vi "getMethods.vi"(0 "reference in":refnum<class "DQMHModuleNode.lvclass">, 5 "error in (no error)":errorcluster) -> (14 "reference out":refnum<class "DQMHModuleNode.lvclass">, 15 "methods":refnum<class "MultiLineString.lvclass">, 19 "error out":errorcluster)   [LabVIEW 2014, in "DQMHModuleNode.lvclass"]
doc: "public MultiLineString getMethods()"
uses:
  <resource>/Framework/Providers/Open_GDS/UML/DQMHModuleNode_class/DQMHModuleNode.lvclass
  <resource>/Framework/Providers/Open_GDS/UML/MultiLineString_class/MultiLineString.lvclass
panel:
  # "Always set\nVI Server class\nto current VI. Do not\nconnect this control\nto the connector pane.\n(Tip!: Just drag\nand drop the icon\ninto the refnum)"
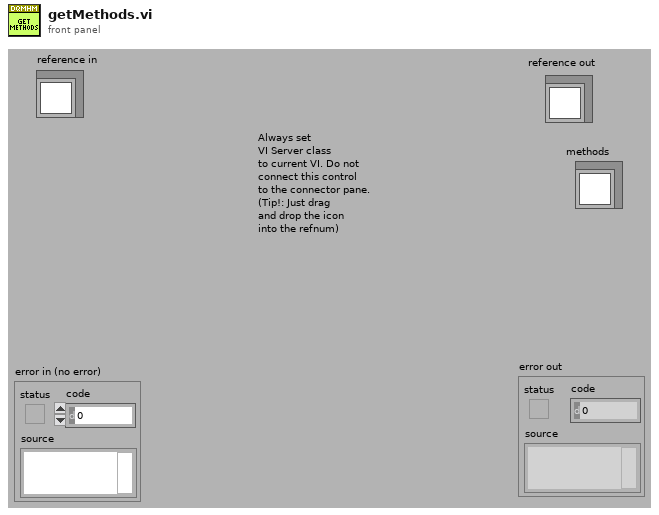
[diagram p1: front panel]
types:
  T1 = typedef "DQMHModuleNode.lvclass/ObjectAttributes.ctl" = cluster{"midHeight":dbl, "botHeight":dbl, "Name":refnum<class "MultiLineString.lvclass">, "Description":refnum<class "MultiLineString.lvclass">, "InternalData":refnum<class "MultiLineString.lvclass">, "Events":refnum<class "MultiLineString.lvclass">, "DEFAULT_COMPARTMENT_HEIGHT":i32, "DEFAULT_WIDTH":i32, "DEFAULT_HEIGHT":i32, "showEvents":bool, "showInternalData":bool, "ClassPath":path, "Template":string, "Icon":u8[][]}
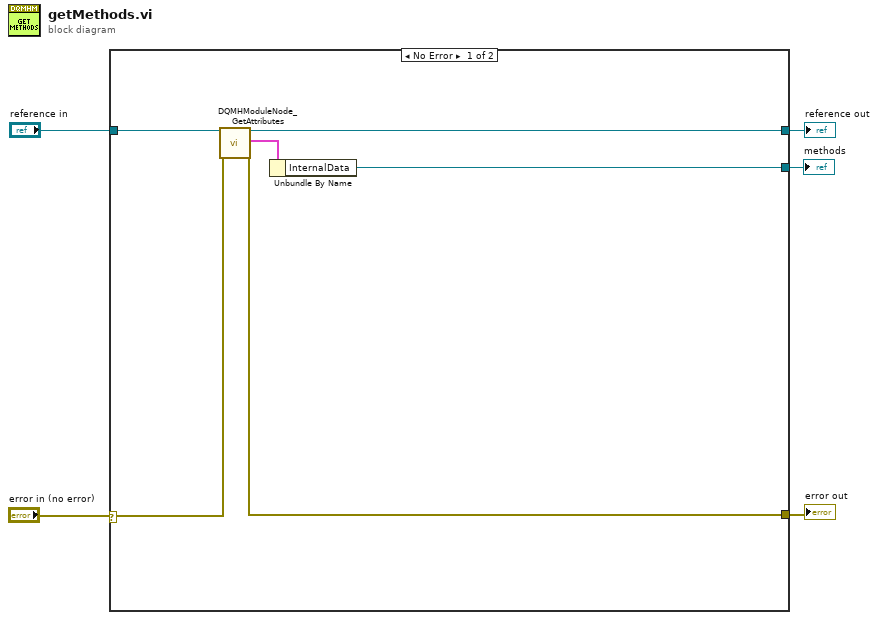
[diagram p0: block diagram]
diagram:
  n1 = case shown="No Error" "error in (no error)" {
    selector: "error in (no error)" -> [w7 w12]
    tunnel: "reference in" -> [w11 w13]
    tunnel: [w10 w12] -> w4
    tunnel: [w9 w13] -> w3
    tunnel: [w8 _] -> w1
    frame No Error {
      n2 = call <resource>:"DQMHModuleNode_GetAttributes.vi"("reference in"=w11, "error in (no error)"=w7) -> ("reference out"=w9:refnum<class "DQMHModuleNode.lvclass">, "Data"=w6:T1, "error out"=w10:errorcluster)  [unwired: 1 in, 14 out]
      n3 = Unbundle By Name(w6) -> ("InternalData"=w8:refnum<class "MultiLineString.lvclass">)
    }
    frame Error {
    }
  }
  "reference out" <- w3
  "error out" <- w4
  "methods" <- w1
